vi "16 pulses TX 8spc.vi"(7 "reset system clock":bool, 9 "IQ_run":bool=TRUE, 10 "PDW input Valid":bool, 11 "array PDW":u64[](array[numeric])=[0, 0, 0, 0]) -> (0 "trig out":bool, 1 "pulse TX status":T1, 2 "output valid":bool, 3 "IQ out":T2[](array[typedef]), 4 "ready for input":bool)   [LabVIEW 2021]
uses:
  <instrlib>/_niInstr/DSP/v1/Shared/Public/IQ Data.ctl
  <instrlib>/_niInstr/Basic Elements/v1/FPGA/Private/Count Up U64.vi
  <instrlib>/_niInstr/Basic Elements/v1/FPGA/Private/Count Up U32.vi
  <instrlib>/_niInstr/Basic Elements/v1/FPGA/niInstr Basic Elements v1 FPGA.lvlib
  <instrlib>/_niInstr/DSP/v1/Shared/niInstr DSP v1 Shared.lvlib
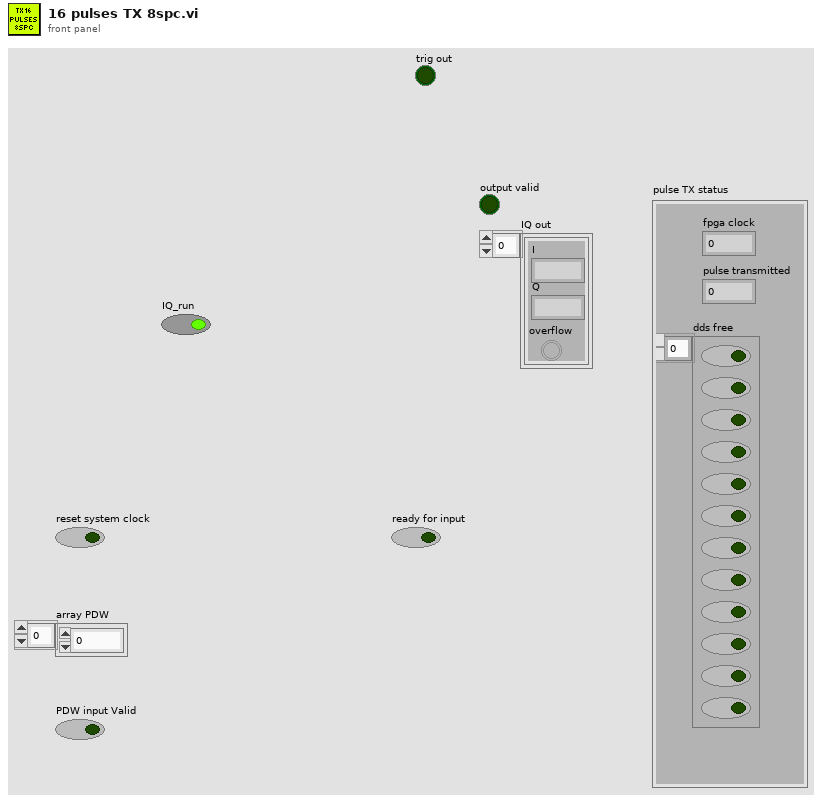
[diagram p1: front panel]
types:
  T1 = cluster{"fpga clock":u64, "pulse transmitted":u32, "dds free":bool[]}
  T2 = typedef "niInstr DSP v1 Shared.lvlib/IQ Data.ctl" = cluster{"I":fxp<+/-,18,1>, "Q":fxp<+/-,18,1>, "overflow":bool}
  T3 = typedef "pdw.ctl" = cluster{"PW":u32, "frequency shift":fxp<+/-,48,0>, "amp":fxp<+/-,18,1>, "mode type":T4, "mode depth":u32, "mode filter":u8, "phase shift":fxp<+/-,16,1>, "pulse shape filter":u8}
  T4 = typedef "mode_type.ctl" = enum8{"CW", "from memory 1", "NC - cw", "LFM", "BPSK", "QPSK"}
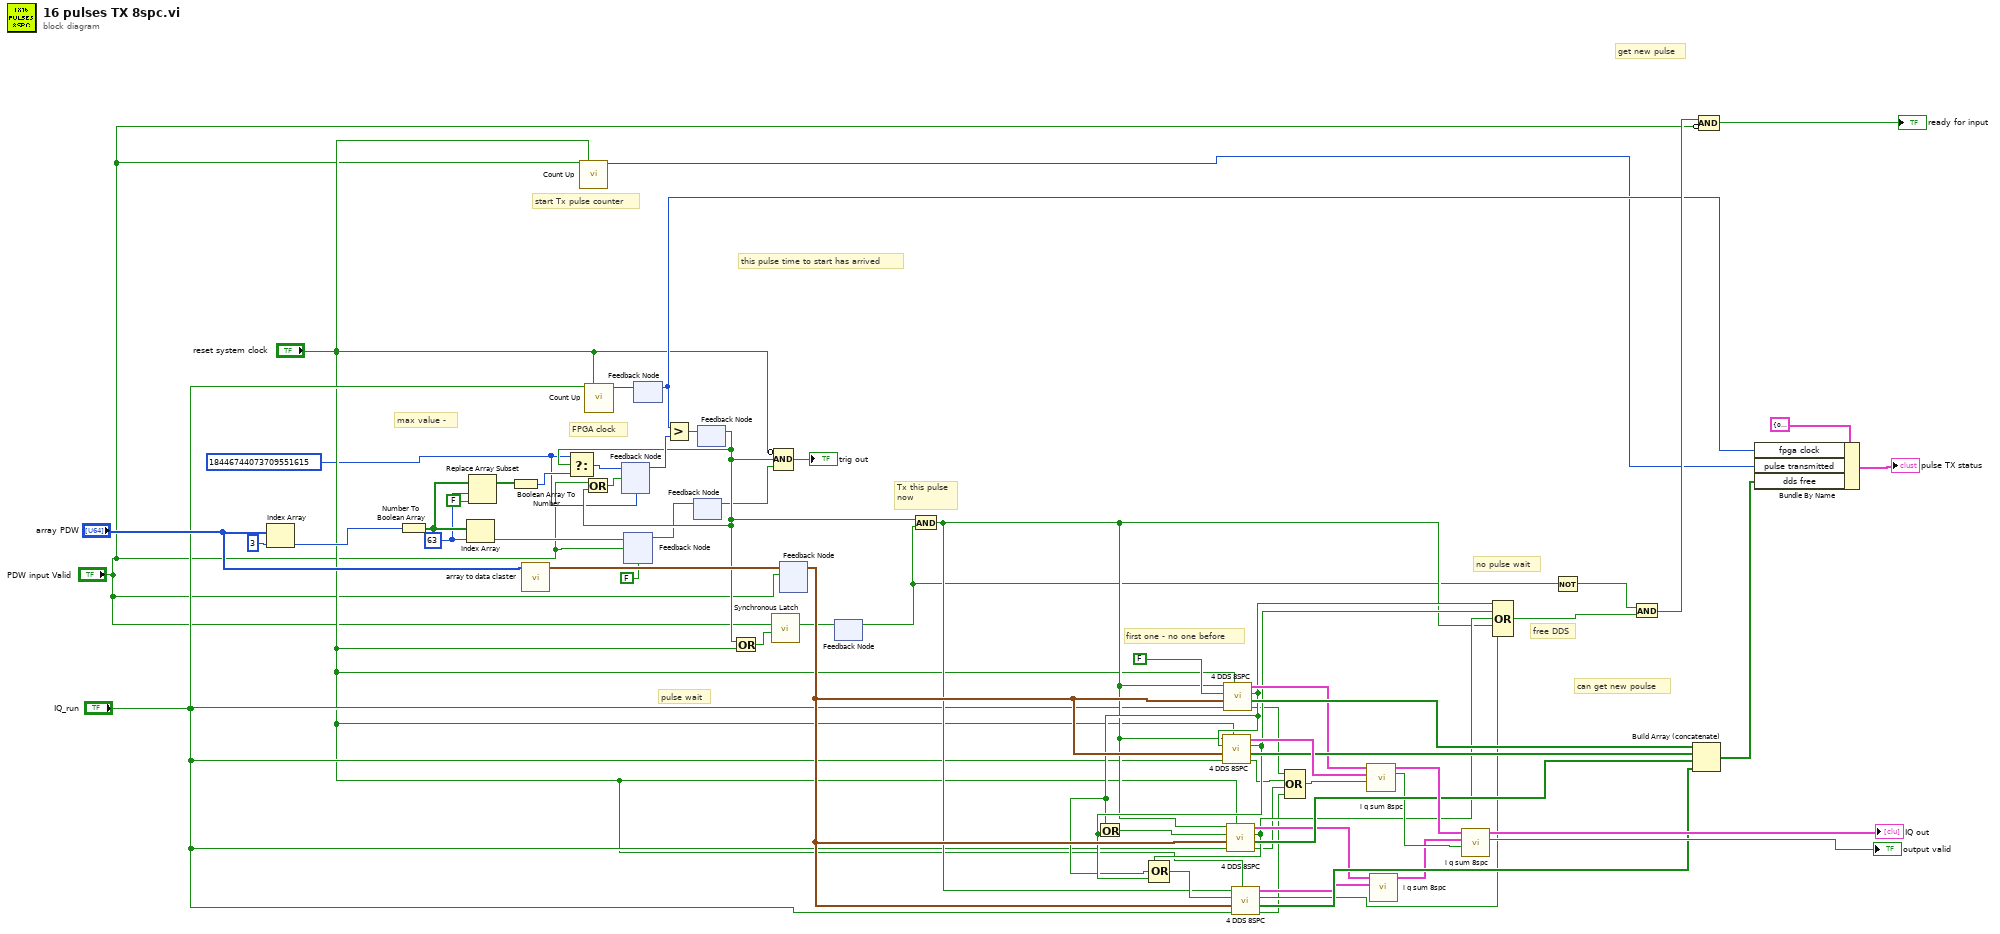
[diagram p0: block diagram]
diagram:
  w13 = 63 ("index")
  w5 = u64 18446744073709551615 ("t")
  # "start Tx pulse counter"
  # "FPGA clock"
  # "this pulse time to start has arrived"
  # "first one - no one before"
  # "max value -"
  # "Tx this pulse\nnow"
  # "get new pulse"
  # "pulse wait"
  # "can get new poulse"
  # "no pulse wait"
  # "free DDS"
  n1 = Index Array(array="array PDW", index=3) -> (element=w15:u64)
  n2 = Number To Boolean Array(number=w15) -> (Boolean array=w14:bool[])
  n3 = Index Array(array=w14, index=w13) -> (element=w9:bool)
  n4 = Replace Array Subset(array=w14, new element=FALSE ("new element/subarray"), index=w13) -> (w11:bool[])
  n5 = Boolean Array To Number(Boolean array=w11) -> (number=w10:u64)
  n6 = call "array to data claster.vi"("Array"="array PDW") -> ("Cluster"=w55:T3)  [unwired: 10 in]
  n7 = call-poly <instrlib>:"Count Up.vi"("increment"="PDW input Valid", "reset"="reset system clock") -> ("count out"=w21:u32)  [unwired: 13 in]
  n8 = call-poly <instrlib>:"Count Up.vi"("increment"="IQ_run", "reset"="reset system clock") -> ("count out"=w54:u64)  [unwired: 13 in]
  n9 = feedback #1(w5) -> (w48:u64)
  n10 = feedback #2(FALSE) -> (w3:bool)
  n11 = feedback-in #2(w9, "PDW input Valid") -> ()
  n12 = feedback #3() -> (w22:u64)  [unwired: 1 in]
  n13 = feedback-in #3(w54) -> ()
  n14 = Greater?(x=w22, y=w48) -> (0:w63:bool)
  n15 = feedback #4() -> (w2:bool)  [unwired: 1 in]
  n16 = feedback-in #4(w3) -> ()
  n17 = feedback #5() -> (w8:bool)  [unwired: 1 in]
  n18 = Select(t=w5, s=w8, f=w10) -> (s? t:f=w52:u64)
  n19 = Or(x="PDW input Valid", y=w8) -> (x .or. y?=w53:bool)
  n20 = feedback-in #1(w52, w53) -> ()
  n21 = feedback-in #5(w63) -> ()
  n22 = Or(x=w8, y="reset system clock") -> (x .or. y?=w18:bool)
  n23 = call <instrlib>:"Synchronous Latch.vi"("clear"=w18, "set"="PDW input Valid") -> ("out"=w17:bool)  [unwired: 9 in]
  n24 = Compound Arithmetic op=AND(invert "reset system clock", w8, w2) -> (→"trig out":bool)
  n25 = feedback #6() -> (w36:T3)  [unwired: 1 in]
  n26 = feedback-in #6(w55, "PDW input Valid") -> ()
  n27 = feedback #7() -> (w16:bool)  [unwired: 1 in]
  n28 = feedback-in #7(w17) -> ()
  n29 = And(x=w8, y=w16) -> (x .and. y?=w30:bool)
  n30 = call "4 DDS 8SPC.vi"("clear DDS"="reset system clock", "input valid"="IQ_run", "pdw in"=w36, "free DDS before me?"=FALSE, "new PDW in"=w30) -> ("output valid"=w27:bool, "state of every DDS"=w47:bool[], "have free DDS"=w32:bool, "IQ out"=w42:T2[])  [unwired: 3 in]
  n31 = call "4 DDS 8SPC.vi"("clear DDS"="reset system clock", "input valid"="IQ_run", "pdw in"=w36, "free DDS before me?"=w32, "new PDW in"=w30) -> ("output valid"=w29:bool, "state of every DDS"=w46:bool[], "have free DDS"=w33:bool, "IQ out"=w59:T2[])  [unwired: 3 in]
  n32 = Or(x=w32, y=w33) -> (x .or. y?=w60:bool)
  n33 = call "4 DDS 8SPC.vi"("clear DDS"="reset system clock", "input valid"="IQ_run", "pdw in"=w36, "free DDS before me?"=w60, "new PDW in"=w30) -> ("output valid"=w26:bool, "state of every DDS"=w45:bool[], "have free DDS"=w31:bool, "IQ out"=w38:T2[])  [unwired: 3 in]
  n34 = Compound Arithmetic op=OR(w31, w32, w33) -> (w34:bool)
  n35 = call "4 DDS 8SPC.vi"("clear DDS"="reset system clock", "input valid"="IQ_run", "pdw in"=w36, "free DDS before me?"=w34, "new PDW in"=w30) -> ("output valid"=w25:bool, "state of every DDS"=w40:bool[], "have free DDS"=w35:bool, "IQ out"=w39:T2[])  [unwired: 3 in]
  n36 = Compound Arithmetic op=OR(w27, w29, w26, w25) -> (w28:bool)
  n37 = call "i q sum 8spc.vi"("input valid"=w28, "IQ in 2"=w59, "IQ in"=w42) -> ("output valid"=w44:bool, "IQ out"=w57:T2[])  [unwired: 7 in]
  n38 = call "i q sum 8spc.vi"("IQ in 2"=w39, "IQ in"=w38) -> ("IQ out"=w37:T2[])  [unwired: 8 in, 1 out]
  n39 = call "i q sum 8spc.vi"("input valid"=w44, "IQ in 2"=w37, "IQ in"=w57) -> ("output valid"=→"output valid":bool, "IQ out"=→"IQ out":T2[])  [unwired: 7 in]
  n40 = Compound Arithmetic op=OR(w32, w33, w31, w30, w35) -> (w56:bool)
  n41 = Not(x=w16) -> (.not. x?=w49:bool)
  n42 = And(x=w49, y=w56) -> (x .and. y?=w50:bool)
  n43 = Build Array (concatenate)(w47, w46, w45, w40) -> (w20:bool[])
  n44 = Compound Arithmetic op=AND(w50, invert "PDW input Valid") -> (→"ready for input":bool)
  n45 = Bundle By Name(cluster=T1 {"fpga clock"=0, "pulse transmitted"=0, "dds free"=[FALSE, FALSE, FALSE, FALSE, FALSE, FALSE, FALSE, FALSE, FALSE, FALSE, FALSE, FALSE, FALSE, FALSE, FALSE, FALSE]} ("pulse TX status"), "fpga clock"=w22, "pulse transmitted"=w21, "dds free"=w20) -> (→"pulse TX status":T1)
